vi "dfd_Group Delay_Decimate Design Info.vi"(8 "error in (no error)":errorcluster, 11 "Group Delay Design Info (in)":T1={"p"=2, "freq grid"=[], "d"=[], "weight"=[], "Order"=0, "radius"=0.0}) -> (0 "error out":errorcluster, 1 "Group Delay Design Info (even)":T1={"p"=2, "freq grid"=[], "d"=[], "weight"=[], "Order"=0, "radius"=0.0}, 2 "Group Delay Design Info (odd)":T1={"p"=2, "freq grid"=[], "d"=[], "weight"=[], "Order"=0, "radius"=0.0}, 3 "Group Delay Design Info (dup)":T1={"p"=2, "freq grid"=[], "d"=[], "weight"=[], "Order"=0, "radius"=0.0})   [LabVIEW 2017, in "NI_DigFilter_Design.lvlib"]
uses:
  <vilib>/addons/Digital Filter Design/NI_DigFilter_Design.lvlib
  <vilib>/addons/Digital Filter Design/_GroupDelay.llb/dfd_Group Delay_Design Info.ctl
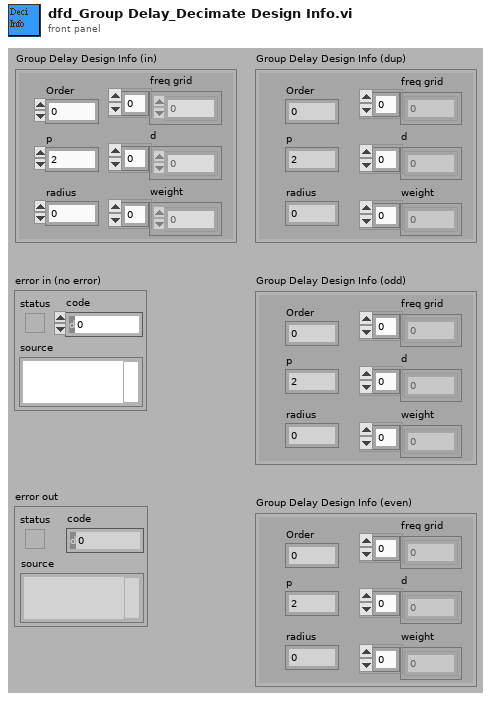
[diagram p1: front panel]
types:
  T1 = typedef "dfd_Group Delay_Design Info.ctl" = cluster{"p":i32, "freq grid":dbl[], "d":dbl[], "weight":dbl[], "Order":i32, "radius":dbl}
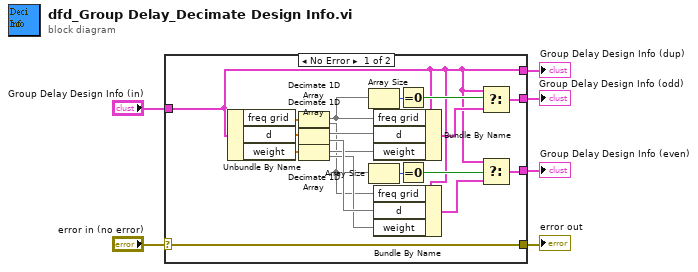
[diagram p0: block diagram]
diagram:
  n1 = case shown="No Error" "error in (no error)" {
    selector: "error in (no error)" -> [w10 w26]
    tunnel: [w10 w26] -> w4
    tunnel: "Group Delay Design Info (in)" -> [w9 _]
    tunnel: [w9 _] -> w1
    tunnel: [w8 _] -> w2
    tunnel: [w7 _] -> w3
    frame No Error {
      n2 = Unbundle By Name(w9) -> ("freq grid"=w25:dbl[], "d"=w24:dbl[], "weight"=w23:dbl[])
      n3 = Decimate 1D Array(w25) -> (w17:dbl[], w18:dbl[])
      n4 = Decimate 1D Array(w24) -> (w22:dbl[], w21:dbl[])
      n5 = Decimate 1D Array(w23) -> (w20:dbl[], w19:dbl[])
      n6 = Array Size(array=w17) -> (size(s)=w16:i32)
      n7 = Array Size(array=w18) -> (size(s)=w15:i32)
      n8 = Bundle By Name(cluster=w9, "freq grid"=w17, "d"=w22, "weight"=w20) -> (w12:T1)
      n9 = Bundle By Name(cluster=w9, "freq grid"=w18, "d"=w21, "weight"=w19) -> (w11:T1)
      n10 = Equal To 0?(x=w16) -> (x = 0?=w14:bool)
      n11 = Equal To 0?(x=w15) -> (x = 0?=w13:bool)
      n12 = Select(t=w9, s=w14, f=w12) -> (s? t:f=w8:T1)
      n13 = Select(t=w9, s=w13, f=w11) -> (s? t:f=w7:T1)
    }
    frame Error {
    }
  }
  "Group Delay Design Info (dup)" <- w1
  "Group Delay Design Info (odd)" <- w2
  "Group Delay Design Info (even)" <- w3
  "error out" <- w4
